vi "Describe Path Failure.vi"(1 "Expected":path, 2 "Got":path) -> (0 "Failure Description":string)   [LabVIEW 2013]
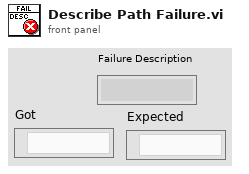
[diagram p1: front panel]
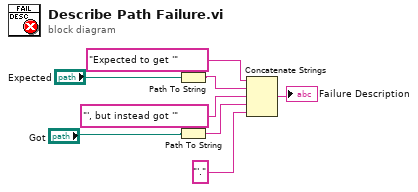
[diagram p0: block diagram]
diagram:
  n1 = Path To String(path="Expected") -> (string=w1:string)
  n2 = Path To String(path="Got") -> (string=w3:string)
  n3 = Concatenate Strings("Expected to get '", w1, "', but instead got '", w3, "'.") -> (→"Failure Description":string)
